vi "ReadWrite.ProcessData.vi"(8 "error in":errorcluster, 10 "timeout ms":i32=100, 11 "ReadWrite in":refnum<class "ReadWrite.lvclass">) -> (0 "error out":errorcluster, 1 "Timeout?":bool, 2 "Values":dbl[](array[numeric]), 3 "ReadWrite out":refnum<class "ReadWrite.lvclass">, 5 "Detect?":bool[](array[boolean]))   [LabVIEW 2024, in "VS Plugin Data Access Engine.lvlib" / "ReadWrite.lvclass"]
uses:
  ReadWrite.lvclass
  ReadWrite.lvclass/ReadWrite.ctl
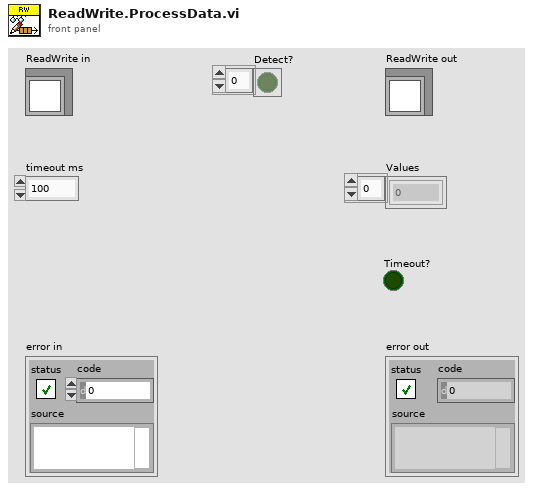
[diagram p1: front panel]
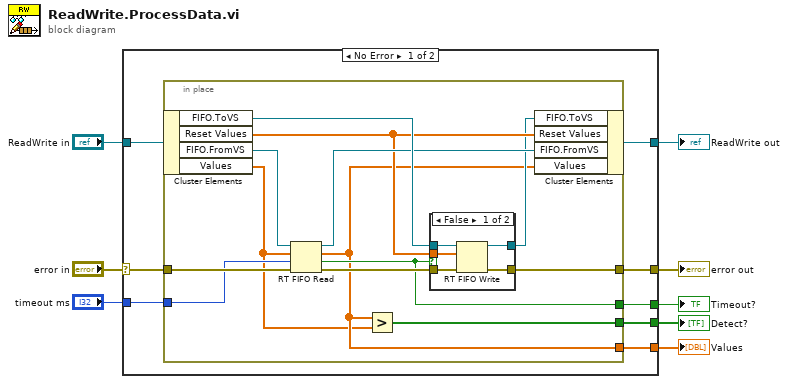
[diagram p0: block diagram]
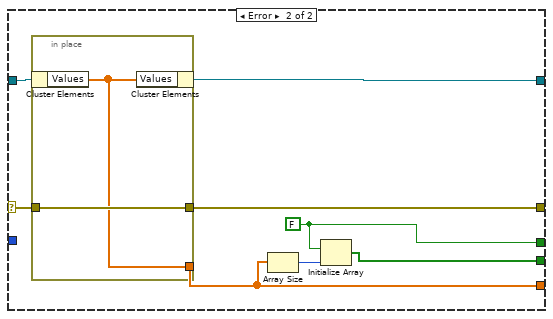
[diagram p3: hidden frame]
diagram:
  n1 = case shown="No Error" "error in" {
    selector: "error in" -> [w16 w43]
    tunnel: [w15 w44] -> w7
    tunnel: [w12 w41] -> w1
    tunnel: "ReadWrite in" -> [w13 w42]
    tunnel: [w14 w39] -> w6
    tunnel: "timeout ms" -> [w11 _]
    tunnel: [w10 w37] -> w4
    tunnel: [w9 w38] -> w3
    frame No Error {
      n2 = in-place {
        in-place-border: w16 -> [w29]
        in-place-border: [w27] -> w15
        in-place-border: [w19] -> w14
        in-place-border: w11 -> [w21]
        in-place-border: [w20] -> w10
        in-place-border: [w17] -> w9
        n3 = in-place-cluster #1(w13) -> ("FIFO.ToVS"=w25:refnum<k33>, "Reset Values"=w23:dbl[], "FIFO.FromVS"=w26:refnum<k33>, "Values"=w18:dbl[])
        n4 = RT FIFO Read(0:w26, 1:w18, 2:w21, 3:w29) -> (8:w24:refnum<k33>, 9:w19:dbl[], 10:w20:bool, 11:w28:errorcluster)  [unwired: 1 out]
        n5 = Greater?(x=w19, y=w18) -> (0:w17:bool[])
        n6 = case shown="False" w20 {
          tunnel: w28 -> [w34 w36]
          tunnel: w23 -> [w32 _]
          tunnel: w25 -> [w31 w35]
          tunnel: [w30 w35] -> w22
          tunnel: [w33 w36] -> w27
          frame False {
            n7 = RT FIFO Write(0:w31, 1:w32, 3:w34) -> (8:w30:refnum<k33>, 11:w33:errorcluster)  [unwired: 2 in, 2 out]
          }
          frame True {
          }
        }
        n8 = in-place-cluster #1("FIFO.ToVS"=w22, "Reset Values"=w23, "FIFO.FromVS"=w24, "Values"=w19) -> (w12:refnum<class "ReadWrite.lvclass">)
      }
    }
    frame Error {
      w37 = FALSE ("empty?")
      n9 = in-place {
        in-place-border: [w45] -> w39
        in-place-border: [w46] -> w44
        in-place-border: w43 -> [w46]
        n10 = in-place-cluster #2(w42) -> ("Values"=w45:dbl[])
        n11 = in-place-cluster #2("Values"=w45) -> (w41:refnum<class "ReadWrite.lvclass">)
      }
      n12 = Array Size(array=w39) -> (size(s)=w40:i32)
      n13 = Initialize Array(w37, w40) -> (w38:bool[])
    }
  }
  "error out" <- w7
  "ReadWrite out" <- w1
  "Values" <- w6
  "Timeout?" <- w4
  "Detect?" <- w3
